vi "Get Apriltag Number from Image.vi"(10 "tag info":T1={"diameter points"={"first point"={"x"=0.0, "y"=0.0}, "projected point"={"x"=0.0, "y"=0.0}}, "normalized center"={"x"=0.0, "y"=0.0}, "Overall Score"=0.0, "Distance (ft)"=0.0, "Offset Angle"=0.0, "Tag corner points"=[], "Tag Center"={"X"=0.0, "Y"=0.0}, "Tag Yaw"=0.0, "Tag Pitch"=0.0, "Target Roll (deg)"=0.0, "AprilTag Number"=68} {"Tag Center"."Y" format="%0.2f"; "Tag Center"."X" format="%0.2f"}, 11 "Image":T2(plugin-control)) -> (1 "Execution Time (msec)":dbl, 2 "tag info out":T1={"diameter points"={"first point"={"x"=0.0, "y"=0.0}, "projected point"={"x"=0.0, "y"=0.0}}, "normalized center"={"x"=0.0, "y"=0.0}, "Overall Score"=0.0, "Distance (ft)"=0.0, "Offset Angle"=569.258018632146, "Tag corner points"=[], "Tag Center"={"X"=0.0, "Y"=0.0}, "Tag Yaw"=0.0, "Tag Pitch"=0.0, "Target Roll (deg)"=0.0, "AprilTag Number"=68} {"Tag Center"."Y" format="%0.2f"; "Tag Center"."X" format="%0.2f"}, 3 "AprilTag#":i32)   [LabVIEW 2023]
uses:
  AprilTag Target Fields.ctl
  <vilib>/vision/NI_Vision_Development_Module.lvlib
panel:
  in  "Range":cluster{"Lower value":sgl, "Upper value":sgl}={"Lower value"=75.0, "Upper value"=255.0}
  out "Apriltag":T2(plugin-control)
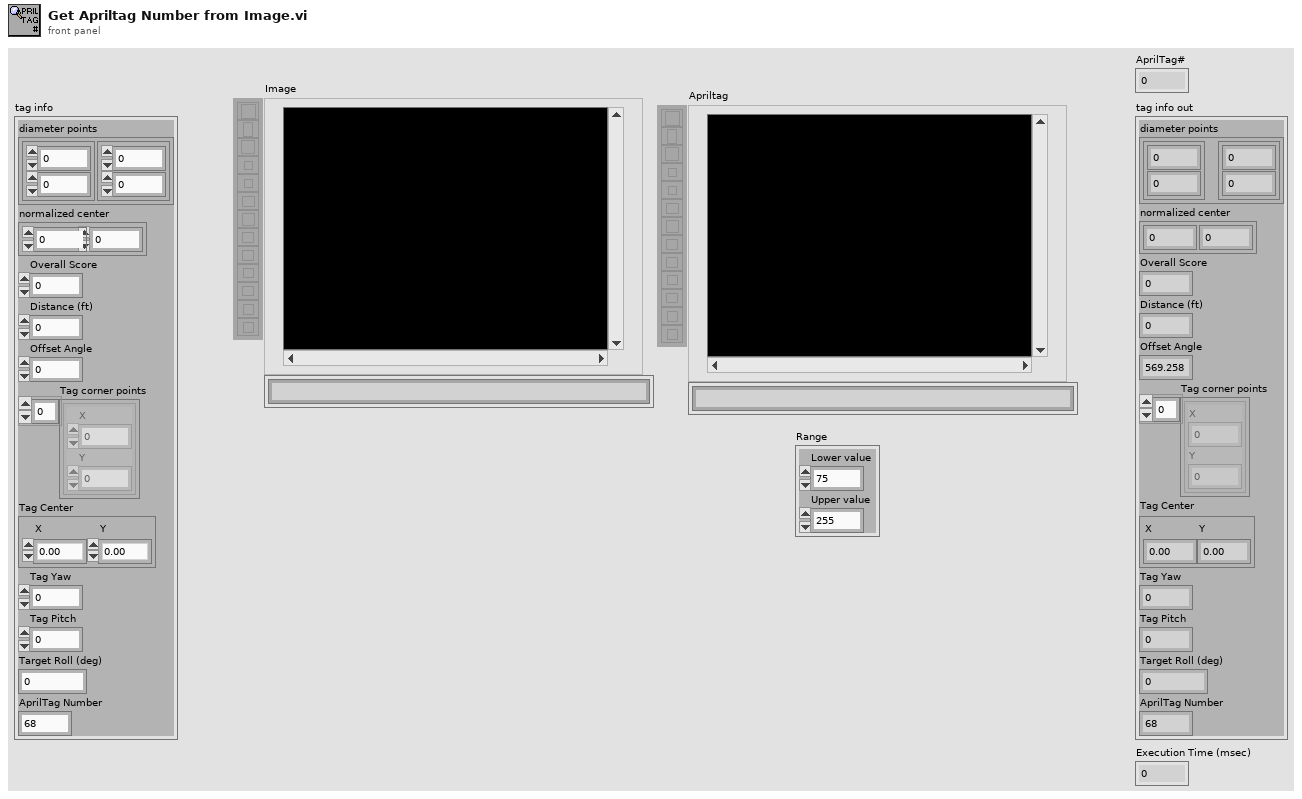
[diagram p1: front panel]
types:
  T1 = typedef "AprilTag Target Fields.ctl" = cluster{"diameter points":cluster{"first point":cluster{"x":dbl, "y":dbl}, "projected point":cluster{"x":dbl, "y":dbl}}, "normalized center":cluster{"x":dbl, "y":dbl}, "Overall Score":dbl, "Distance (ft)":dbl, "Offset Angle":dbl, "Tag corner points":cluster{"X":dbl, "Y":dbl}[], "Tag Center":cluster{"X":dbl, "Y":dbl}, "Tag Yaw":dbl, "Tag Pitch":dbl, "Target Roll (deg)":dbl, "AprilTag Number":i32}
  T2 = typedef "IMAQ Image.ctl" = refnum<image>
  T3 = typedef "Image Type" = u32
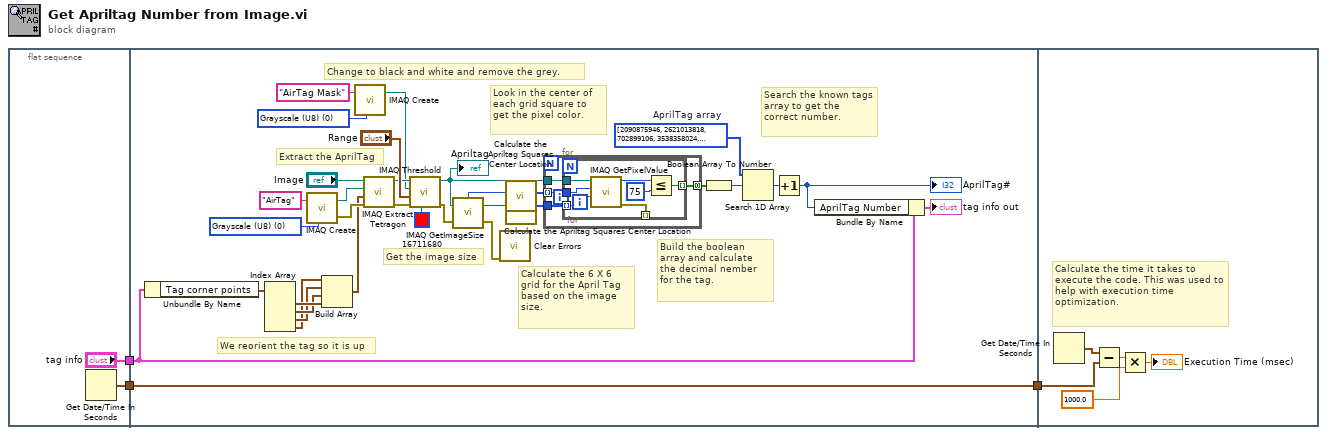
[diagram p0: block diagram]
diagram:
  n1 = flat-sequence {
    tunnel: [w5] -> w2
    tunnel: ["tag info"] -> w1
    tunnel: [w25] -> w3
    tunnel: w2 -> [w25]
    tunnel: w1 -> [w24]
    tunnel: w3 -> [w52]
    frame #0 {
      n2 = Get Date/Time In Seconds() -> (seconds since 1Jan1904=w5:timestamp)
    }
    frame #1 {
      w8 = T3 0 items=["Grayscale (U8)", "Grayscale (I16)", "Grayscale (SGL)", "Complex (CSG)", "RGB (U32)", "HSL (U32)", "RGB (U64)", "Grayscale (U16)"] ("Image Type")
      w32 = T3 0 items=["Grayscale (U8)", "Grayscale (I16)", "Grayscale (SGL)", "Complex (CSG)", "RGB (U32)", "HSL (U32)", "RGB (U64)", "Grayscale (U16)"] ("Image Type")
      w34 = u32[] [2090875946, 2621013818, 702899106, 3538358024, 1663594000, 2908175739, 3842209527, 1632389581, 469213657, 154307819, 610517857, 3321664829, 2540025641, 780983953, 3474046093, 2055835671, 1884137891, 4040607285, 216557965, 1333074778, 3211662662, 103108830]  # AprilTag array
      # "Change to black and white and remove the grey."
      # "Extract the AprilTag"
      # "Get the image size"
      # "Calculate the 6 X 6 grid for the April Tag based on the image size."
      # "Look in the center of each grid square to get the pixel color."
      # "Build the boolean array and calculate the decimal nember for the tag."
      # "Search the known tags array to get the correct number."
      # "We reorient the tag so it is up"
      n3 = Unbundle By Name(w24) -> ("Tag corner points"=w19:cluster{"X":dbl, "Y":dbl}[])
      n4 = Index Array(array=w19) -> (element #1=w23:cluster{"X":dbl, "Y":dbl}, element #2=w22:cluster{"X":dbl, "Y":dbl}, element #3=w21:cluster{"X":dbl, "Y":dbl}, element #4=w20:cluster{"X":dbl, "Y":dbl})  [unwired: 4 in]
      n5 = call "IMAQ Create"("Image Name"="AirTag" ("string"), "Image Type"=w32) -> ("New Image"=w31:T2, "error out"=w30:errorcluster)  [unwired: 2 in, 1 out]
      n6 = Build Array(w20, w21, w22, w23) -> (w18:cluster{"X":dbl, "Y":dbl}[])
      n7 = call "IMAQ Create"("Image Name"="AirTag Mask" ("string"), "Image Type"=w8) -> ("New Image"=w6:T2)  [unwired: 2 in, 2 out]
      n8 = call-poly "IMAQ Extract Tetragon"("error in (no error)"=w30, "Tetragon"=w18, "Image Dst"=w31, "Image Src"="Image") -> ("error out"=w29:errorcluster, "Image Dst Out"=w10:T2)  [unwired: 6 in]
      n9 = call "IMAQ Threshold"("Replace Value"=u32 16711680, "Range"="Range", "Image Dst"=w6, "Image Src"=w10) -> ("Image Dst Out"=w11:T2)  [unwired: 6 in, 1 out]
      "Apriltag" <- w11
      n10 = call "IMAQ GetImageSize"("Image"=w11, "error in (no error)"=w29) -> ("Y Resolution"=w12:i32, "X Resolution"=w16:i32, "error out"=w13:errorcluster)  [unwired: 2 in]
      n11 = call <vilib>:"Clear Errors.vi"("error in (no error)"=w13) -> ()  [unwired: 5 in, 2 out]
      n12 = call "Calculate the Apriltag Squares Center Location.vi"("Pixels"=w16) -> ("Array 2"=w15:i32[])  [unwired: 10 in]
      n13 = call "Calculate the Apriltag Squares Center Location.vi"("Pixels"=w12) -> ("Array 2"=w14:i32[])  [unwired: 10 in]
      n14 = for {
        tunnel: w11 -> [w41]
        tunnel: w15 -> [w40] mode=indexing
        tunnel: w14 -> [w39]
        tunnel: [w38] -> w37 mode=concatenating
        n15 = for {
          tunnel: w41 -> [w48]
          tunnel: [w44] -> w38 mode=indexing
          tunnel: w40 -> [w47]
          tunnel: w39 -> [w46] mode=indexing
          tunnel: [w42] -> _ mode=indexing
          n16 = call "IMAQ GetPixelValue"("Image"=w48, "X Coordinate"=w47, "Y Coordinate"=w46) -> ("Pixel Value (U8)"=w43:u8, "error out"=w42:errorcluster)  [unwired: 3 in, 3 out]
          n17 = Less Or Equal?(x=w43, y=u8 75) -> (x <= y?=w44:bool)
        }
      }
      n18 = Boolean Array To Number(Boolean array=w37) -> (number=w36:u32)
      n19 = Search 1D Array(1D array=w34, element=w36) -> (index of element=w35:i32)  [unwired: 1 in]
      n20 = Increment(x=w35) -> (x+1=w27:i32)
      "AprilTag#" <- w27
      n21 = Bundle By Name(cluster=w24, "AprilTag Number"=w27) -> (→"tag info out":T1)
    }
    frame #2 {
      # "Calculate the time it takes to execute the code. This was used to help with execution time optimization."
      n22 = Get Date/Time In Seconds() -> (seconds since 1Jan1904=w53:timestamp)
      n23 = Subtract(x=w53, y=w52) -> (x-y=w51:dbl)
      n24 = Multiply(x=w51, y=1000.0) -> (x*y=→"Execution Time (msec)":dbl)
    }
  }
